vi "Edit gplugin data file.vi"(0 "Path":path=path "D:/EXP/ABC/ABC.gplugindata", 5 "Lib Name":string, 7 "VI Name":string, 11 "error in (no error)":errorcluster) -> (15 "error out":errorcluster)   [LabVIEW 2021, in "G Plug-in Migrator.lvlib"]
uses:
  G Plug-in Migrator.lvlib
  <vilib>/xml/Load XML String.vi
  <vilib>/xml/Close Reference(Node).vi
  <vilib>/xml/NI_XML.lvlib
  <resource>/objmgr/DOMUserDefRef.rc
  Migrator Reusables/Migrator Reusables.lvlib
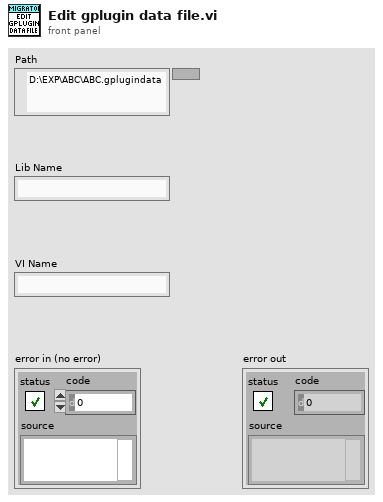
[diagram p1: front panel]
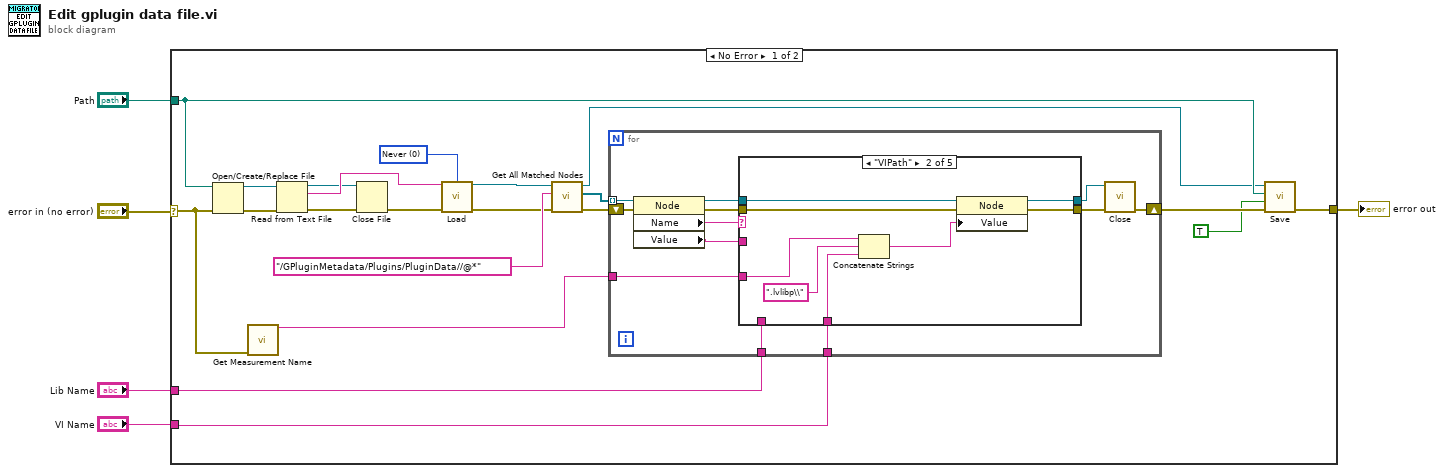
[diagram p0: block diagram]
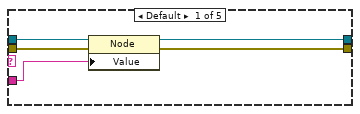
[diagram p2: hidden frame]
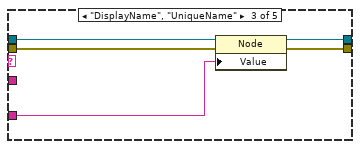
[diagram p3: hidden frame]
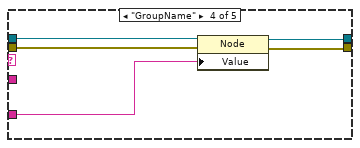
[diagram p4: hidden frame]
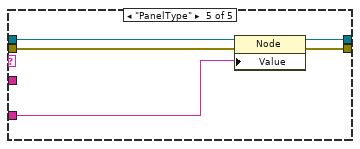
[diagram p5: hidden frame]
diagram:
  n1 = case shown="No Error" "error in (no error)" {
    selector: "error in (no error)" -> [w7 w67]
    tunnel: [w10 w67] -> w5
    tunnel: "Path" -> [w19 _]
    tunnel: "Lib Name" -> [w9 _]
    tunnel: "VI Name" -> [w8 _]
    frame No Error {
      w23 = 0 items=["Never", "Always", "Auto"] ("validate on load (Auto)")
      n2 = Open/Create/Replace File(file path (use dialog)=w19, error in=w7) -> (refnum out=w26:refnum<file>, error out=w24:errorcluster)  [unwired: 4 in, 1 out]
      n3 = call "Get Measurement Name.vi"("error in (no error)"=w7) -> ("Name Out"=w6:string)  [unwired: 13 in, 1 out]
      n4 = Read from Text File(file (use dialog)=w26, error in=w24) -> (refnum out=w16:refnum<file>, text=w25:string, error out=w14:errorcluster)  [unwired: 2 in, 1 out]
      n5 = Close File(refnum=w16, error in=w14) -> (error out=w15:errorcluster)  [unwired: 1 out]
      n6 = call-poly <vilib>:"Load.vi"("XML string"=w25, "validate on load (Auto)"=w23, "error in (no error)"=w15) -> ("DOM document out"=w22:refnum<k20>, "error out"=w12:errorcluster)  [unwired: 10 in, 1 out]
      n7 = call <vilib>:"Get All Matched Nodes.vi"("error in (no error)"=w12, "XPath expression"="/GPluginMetadata/Plugins/PluginData//@*", "node in"=w22) -> ("error out"=w11:errorcluster, "node result array"=w21:refnum<k20>[], "node out"=w13:refnum<k20>)  [unwired: 6 in]
      n8 = for {
        tunnel: w21 -> [w38] mode=indexing
        shift-right: [w33] -> w18
        shift-left: w11 -> [w36]
        tunnel: w9 -> [w29]
        tunnel: w8 -> [w28]
        tunnel: w6 -> [w27]
        n9 = property class="Node"(reference=w38, error in=w36) -> (reference out=w37:refnum<k20>, error out=w35:errorcluster, "Name"=w31:string, "Value"=w30:string)
        n10 = case shown="\"VIPath\"" w31 {
          tunnel: w37 -> [w43 w51 w56 w60 w66]
          tunnel: w35 -> [w40 w48 w55 w61 w64]
          tunnel: [w42 w50 w54 w58 w65] -> w34
          tunnel: [w41 w49 w53 w59 w63] -> w32
          tunnel: w30 -> [w39 _ _ _ _]
          tunnel: w29 -> [_ _ _ _ _]
          tunnel: w28 -> [_ w45 _ _ _]
          tunnel: w27 -> [_ w44 w52 w57 w62]
          frame Default {
            n11 = property class="Node"(reference=w43, error in=w40, "Value"=w39) -> (reference out=w42:refnum<k20>, error out=w41:errorcluster)
          }
          frame "VIPath" {
            n12 = Concatenate Strings(w44, ".lvlibp\\" ("string"), w45) -> (w47:string)
            n13 = property class="Node"(reference=w51, error in=w48, "Value"=w47) -> (reference out=w50:refnum<k20>, error out=w49:errorcluster)
          }
          frame "DisplayName", "UniqueName" {
            n14 = property class="Node"(reference=w56, error in=w55, "Value"=w52) -> (reference out=w54:refnum<k20>, error out=w53:errorcluster)
          }
          frame "GroupName" {
            n15 = property class="Node"(reference=w60, error in=w61, "Value"=w57) -> (reference out=w58:refnum<k20>, error out=w59:errorcluster)
          }
          frame "PanelType" {
            n16 = property class="Node"(reference=w66, error in=w64, "Value"=w62) -> (reference out=w65:refnum<k20>, error out=w63:errorcluster)
          }
        }
        n17 = call-poly <vilib>:"Close.vi"("error in (no error)"=w32, "node"=w34) -> ("error out"=w33:errorcluster)  [unwired: 7 in]
      }
      n18 = call <vilib>:"Save.vi"("error in (no error)"=w18, "overwrite file (True)"=TRUE, "XML file path"=w19, "DOM document in"=w13) -> ("error out"=w10:errorcluster)  [unwired: 5 in, 2 out]
    }
    frame Error {
    }
  }
  "error out" <- w5
